vi "Write IGObjectFactory.vi"(10 "IGObjectFactory":refnum<class "IGObjectFactory.lvclass">, 11 "Search in":refnum<class "Search.lvclass">) -> (3 "Search out":refnum<class "Search.lvclass">)   [LabVIEW 2016, in "Search.lvclass"]
uses:
  Search.lvclass
  IGObjectFactory/IGObjectFactory.lvclass
  Search.lvclass/Search.ctl
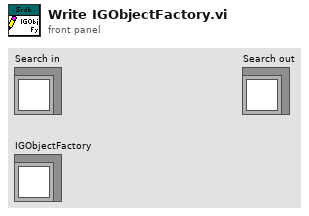
[diagram p1: front panel]
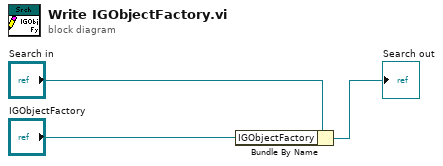
[diagram p0: block diagram]
diagram:
  n1 = Bundle By Name(cluster="Search in", "IGObjectFactory"="IGObjectFactory") -> (→"Search out":refnum<class "Search.lvclass">)
